vi "deleteAllMarkers.vi"   [LabVIEW 2014]
uses:
  <userlib>/Nanonis Prog Interface V5/Nanonis Prog Interface.lvlib
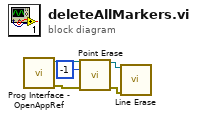
[diagram p0: block diagram]
diagram:
  n1 = call <userlib>:"Prog Interface - OpenAppRef.vi"() -> ("Error out"=w5:errorcluster, "Application reference"=w4:refnum<vi>)  [unwired: 6 in]
  n2 = call <userlib>:"Point Erase.vi"("Application ref in"=w4, "Point index (-1=All points)"=-1, "error in (no error)"=w5) -> ("Application ref out"=w2:refnum<vi>, "error out"=w1:errorcluster)  [unwired: 11 in]
  n3 = call <userlib>:"Line Erase.vi"("Application ref in"=w2, "error in (no error)"=w1) -> ()  [unwired: 12 in, 2 out]
